vi "serialization test.vi"() -> (0 "no error":errorcluster, 1 "name ok":bool, 2 "keys ok":bool, 3 "class identical":bool, 5 "version ok":bool)   [LabVIEW 2013, in "TBM Tests.lvlib"]
uses:
  TBM Tests.lvlib
  root configuration/TBM configuration.lvclass
  <vilib>/NI/Configuration Framework/serializable configuration/NISE_CEF_serializable configuration.lvclass/NISE_CEF_serializable configuration.ctl
  <vilib>/Utility/LVClass/Get LV Class Name.vi
  <vilib>/NI/Configuration Framework/error generator/NISE_error generator.vi
  <vilib>/NI/Configuration Framework/serializable configuration/NISE_CEF_serializable configuration.lvclass
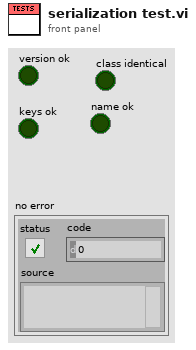
[diagram p1: front panel]
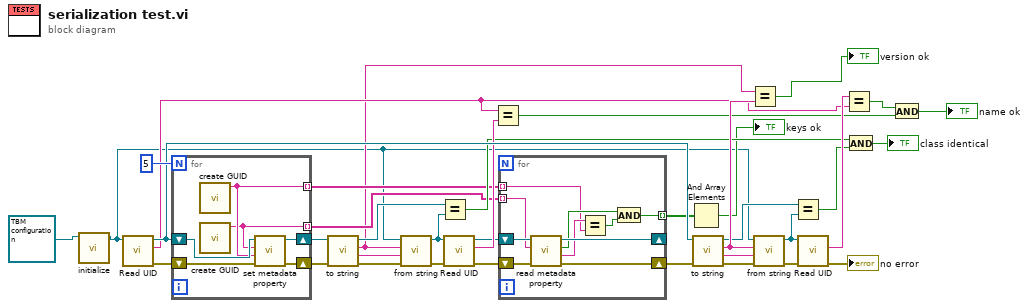
[diagram p0: block diagram]
diagram:
  n1 = call <vilib>:"initialize.vi"("configuration in"=refnum<class "TBM configuration.lvclass"> refnum ("configuration")) -> ("configuration out"=w2:refnum<class "TBM configuration.lvclass">)  [unwired: 8 in, 2 out]
  n2 = call <vilib>:"Read UID.vi"("configuration in"=w2) -> ("error out"=w29:errorcluster, "instance id"=w21:string, "configuration out"=w30:refnum<class "TBM configuration.lvclass">)  [unwired: 8 in]
  n3 = for {
    N: 5 -> [_]
    shift-right: [w42] -> w20
    shift-left: w30 -> [w43]
    shift-right: [w41] -> w26
    shift-left: w29 -> [w40]
    tunnel: [w39] -> w10 mode=indexing
    tunnel: [w38] -> w11 mode=indexing
    n4 = call <vilib>:"create GUID.vi"() -> ("uuid"=w39:string)  [unwired: 10 in, 1 out]
    n5 = call <vilib>:"create GUID.vi"() -> ("uuid"=w38:string)  [unwired: 10 in, 1 out]
    n6 = call <vilib>:"set metadata property.vi"("error in"=w40, "value"=w39, "key"=w38, "configuration in"=w43) -> ("error out"=w41:errorcluster, "configuration out"=w42:refnum<class "TBM configuration.lvclass">)  [unwired: 6 in]
  }
  n7 = call-dynamic "to string.vi"("error in"=w26, "configuration in"=w20) -> ("error out"=w27:errorcluster, "data"=w28:string, "version"=w4:string, "configuration out"=w17:refnum<class "TBM configuration.lvclass">)  [unwired: 6 in]
  n8 = call-dynamic "from string.vi"("error in"=w27, "data"=w28, "version"=w4, "configuration in"=w2) -> ("error out"=w23:errorcluster, "configuration out"=w19:refnum<class "TBM configuration.lvclass">)  [unwired: 6 in]
  n9 = Equal?(x=w17, y=w19) -> (x = y?=w12:bool)
  n10 = call <vilib>:"Read UID.vi"("error in"=w23, "configuration in"=w19) -> ("error out"=w8:errorcluster, "instance id"=w22:string, "configuration out"=w9:refnum<class "TBM configuration.lvclass">)  [unwired: 7 in]
  n11 = Equal?(x=w21, y=w22) -> (x = y?=w15:bool)
  n12 = for {
    tunnel: w11 -> [w49] mode=indexing
    tunnel: w10 -> [w46] mode=indexing
    shift-right: [w51] -> _
    shift-left: w9 -> [w52]
    shift-right: [w50] -> w7
    shift-left: w8 -> [w53]
    tunnel: [w44] -> w6 mode=indexing
    n13 = call <vilib>:"read metadata property.vi"("error in"=w53, "key"=w49, "configuration in"=w52) -> ("error out"=w50:errorcluster, "value"=w47:string, "found"=w48:bool, "configuration out"=w51:refnum<class "TBM configuration.lvclass">)  [unwired: 5 in]
    n14 = Equal?(x=w47, y=w46) -> (x = y?=w45:bool)
    n15 = And(x=w48, y=w45) -> (x .and. y?=w44:bool)
  }
  n16 = And Array Elements(Boolean array=w6) -> (logical AND=→"keys ok":bool)
  n17 = call-dynamic "to string.vi"("error in"=w7, "configuration in"=w30) -> ("error out"=w37:errorcluster, "data"=w32:string, "version"=w36:string, "configuration out"=w18:refnum<class "TBM configuration.lvclass">)  [unwired: 6 in]
  n18 = Equal?(x=w4, y=w36) -> (x = y?=→"version ok":bool)
  n19 = call-dynamic "from string.vi"("error in"=w37, "data"=w32, "version"=w36, "configuration in"=w2) -> ("error out"=w35:errorcluster, "configuration out"=w16:refnum<class "TBM configuration.lvclass">)  [unwired: 6 in]
  n20 = Equal?(x=w18, y=w16) -> (x = y?=w13:bool)
  n21 = call <vilib>:"Read UID.vi"("error in"=w35, "configuration in"=w16) -> ("error out"=→"no error":errorcluster, "instance id"=w33:string)  [unwired: 7 in, 1 out]
  n22 = Equal?(x=w33, y=w21) -> (x = y?=w24:bool)
  n23 = And(x=w12, y=w13) -> (x .and. y?=→"class identical":bool)
  n24 = And(x=w24, y=w15) -> (x .and. y?=→"name ok":bool)
